vi "PH_Sequencer.set MA MM1.vi"(0 "i ref in":refnum<vi>, 2 "High Energy Position?":bool, 5 "error in":errorcluster) -> (14 "i ref out":refnum<vi>, 19 "error out":errorcluster)   [LabVIEW 2014, in "PH_Sequencer.lvlib"]
uses:
  PH_Sequencer.lvlib
  PH_4_Pos_Selector/PH_4_Pos_Selector.Position Selector.ctl
  PH_Beamline/PH_Beamline.6P 4 Pos Selector Instances.ctl
  PH_4_Pos_Selector/PH_4_Pos_Selector.lvlib
  PH_Beamline/PH_Beamline.lvlib
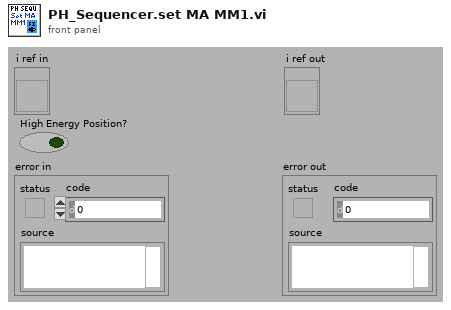
[diagram p1: front panel]
types:
  T1 = typedef "PH_4_Pos_Selector.lvlib/PH_4_Pos_Selector.Position Selector.ctl" = u16
  T2 = typedef "PH_Beamline.lvlib/PH_Beamline.6P 4 Pos Selector Instances.ctl" = string
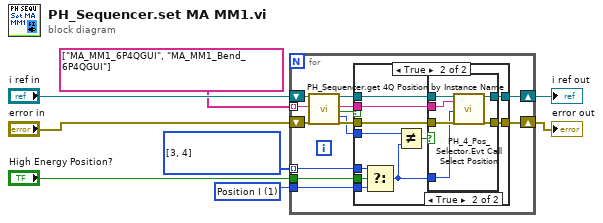
[diagram p0: block diagram]
diagram:
  w1 = T1[] [3, 4] items=["unknown", "Position I", "Position II", "Position III", "Position IV", "moving"]
  w3 = T1 1 items=["unknown", "Position I", "Position II", "Position III", "Position IV", "moving"] ("Wanted Position")
  n1 = for {
    tunnel: T2[] ["MA_MM1_6P4QGUI", "MA_MM1_Bend_6P4QGUI"] -> [w14] mode=indexing
    tunnel: "High Energy Position?" -> [w13]
    tunnel: w1 -> [w10] mode=indexing
    tunnel: w3 -> [w9]
    shift-right: [w18] -> w7
    shift-left: "error in" -> [w12]
    shift-right: [w19] -> w8
    shift-left: "i ref in" -> [w11]
    n2 = call "PH_Sequencer.get 4Q Position by Instance Name.vi"("VI in"=w11, "Wanted 4Q Instance"=w14, "error in"=w12) -> ("VI out"=w21:refnum<vi>, "Instancename"=w17:string, "linked"=w16:bool, "Current Position"=w15:T1, "error out"=w20:errorcluster)  [unwired: 11 in, 1 out]
    n3 = case shown="True" w16 {
      tunnel: w21 -> [w23 w34]
      tunnel: w20 -> [w22 w33]
      tunnel: w17 -> [_ w32]
      tunnel: [w23 w31] -> w19
      tunnel: [w22 w30] -> w18
      tunnel: w15 -> [_ w29]
      tunnel: w13 -> [_ w26]
      tunnel: w10 -> [_ w25]
      tunnel: w9 -> [_ w24]
      frame False {
      }
      frame True {
        n4 = Select(t=w25, s=w26, f=w24) -> (s? t:f=w28:T1)
        n5 = Not Equal?(x=w29, y=w28) -> (x != y?=w27:bool)
        n6 = case shown="True" w27 {
          tunnel: w34 -> [w36 w42]
          tunnel: w33 -> [w35 w41]
          tunnel: w32 -> [_ w40]
          tunnel: [w36 w39] -> w31
          tunnel: [w35 w38] -> w30
          tunnel: w28 -> [_ w37]
          frame False {
          }
          frame True {
            n7 = call "PH_4_Pos_Selector.Evt Call Select Position.vi"("i ref in"=w42, "4 Pos instance"=w40, "Wanted Position"=w37, "error in"=w41) -> ("i ref out"=w39:refnum<vi>, "error out"=w38:errorcluster)  [unwired: 14 in]
          }
        }
      }
    }
  }
  "i ref out" <- w8
  "error out" <- w7
